vi "Main Page.vi"(8 "error in (no error)":errorcluster, 11 "Node Ptr":T1 format="%.0x") -> (0 "error out":errorcluster)   [LabVIEW 2020, in "Protection and Counter Addon System Explorer.lvlib"]
uses:
  Protection and Counter Addon System Explorer.lvlib
  <vilib>/NI VeriStand/Custom Device API/Custom Device Item Ref.ctl
  <vilib>/NI/NI VeriStand Hardware Resource Discovery/_Types/Filter Type.ctl
  Addon Shared/Types/986x.ctl
  Addon Shared/SubVIs/GUID Lookup.vi
  <vilib>/NI VeriStand/Custom Device API/NI VeriStand - Get Item Property.vi
  <vilib>/NI VeriStand/Custom Device API/Get Item Property (Boolean).vi
  <vilib>/NI VeriStand/Custom Device API/Get Item Property (String).vi
  <vilib>/NI VeriStand/Custom Device API/Get Item Property (Dependent File).vi
  <vilib>/NI VeriStand/Custom Device API/Get Item Property (U32).vi
  <vilib>/NI VeriStand/Custom Device API/Get Item Property (String Array).vi
  <vilib>/NI VeriStand/Custom Device API/Custom Device API.lvlib
  <vilib>/NI/NI VeriStand Hardware Resource Discovery/NIVS Hardware Discovery.lvlib
  Addon Shared/Protection and Counter Addon Shared.lvlib
  SubModules/985x-Support/Source/System Explorer/985x Support System Explorer.lvlib
panel:
  in  "Header":cluster{"Section Name":string}={"Section Name"="Addon Settings"}
  in  "Tab Control":enum32{"Main Setting", "FPGA Settings"}(tab)
  in  "FD ISO Mode":u32(ring) items=["ISO", "Non ISO", "ISO Legacy"]
  in  "Description":string
  in  "Name":string
  out "Version":string
  in  "Port":string
  in  "CAN Browse":bool
  out "XNET Database":refnum<k21>
  out "XNET Cluster":refnum<k21>
  out "I/O Mode":u32(ring) items=["CAN 2.0", "CAN FD", "CAN FD+BRS"]
  in  "Baud Rate":u64
  in  "Termination":enum16{"Off", "On"}(ring)
  in  "FD Baud Rate":u64
  in  "Use Legacy":bool
  in  "Loop Priority":i32=100 format="%.0p"
  in  "985x Chn":u16(ring) caption="Channel Number"
  in  "Use 985x":bool
  in  "Enable Bitfile":bool
  in  "Bitfile Path":path caption="Bitfile Path (Browse the bitfile to check if it supports 985x.)"
  in  "RIO Device":string
  in  "RIO Browse":bool
  in  "SHDocVw.IWebBrowser2":refnum<k7>(container)
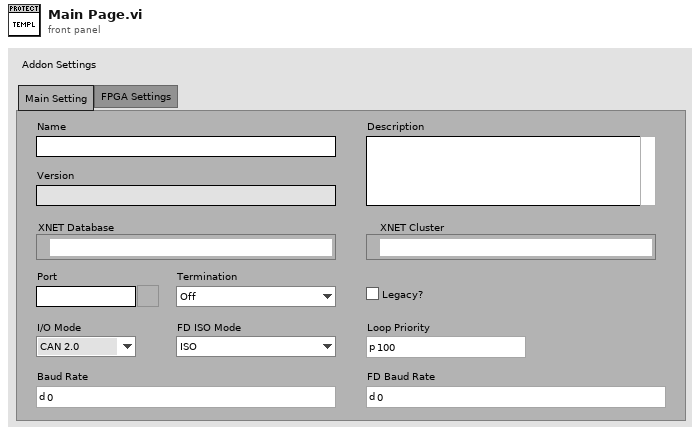
[diagram p1: front panel]
types:
  T1 = typedef "Custom Device API.lvlib/Custom Device Item Ref.ctl" = u64
  T2 = typedef "Protection and Counter Addon Shared.lvlib/986x.ctl" = cluster{"Enable":bool, "RIO Device":string, "Bitfile":path, "985x Valid":bool, "Use 985x":bool, "Channel Number":u32, "Valid Channels":string[]}
  T3 = typedef "Protection and Counter Addon Shared.lvlib/XNET Settings.ctl" = cluster{"Database":refnum<k21>, "Cluster":refnum<k21>, "Port":string, "Baud rate [Bd]":u64, "Termination":u32, "CAN I/O Mode":u32, "FD Baud rate [Bd]":u64, "Priority":i32, "Use Legacy":bool, "FD ISO Mode":u32}
  T4 = typedef "Custom Device API.lvlib/Custom Device Item Info.ctl" = cluster{"Name":string, "Is Channel":bool, "GUID":string, "Is Waveform":bool}
  T5 = typedef "NIVS Hardware Discovery.lvlib/Filter Type.ctl" = enum16{"Device Category", "Product Name", "Ethernet", "XNET", "VISA", "FPGA", "EtherCAT Master", "DAQmx", "GPIB", "Serial"}
  T6 = typedef "Custom Device API.lvlib/Custom Device Commands.ctl" = enum16{"Default", "Item renamed", "Shutdown", "Dynamic button pressed"}
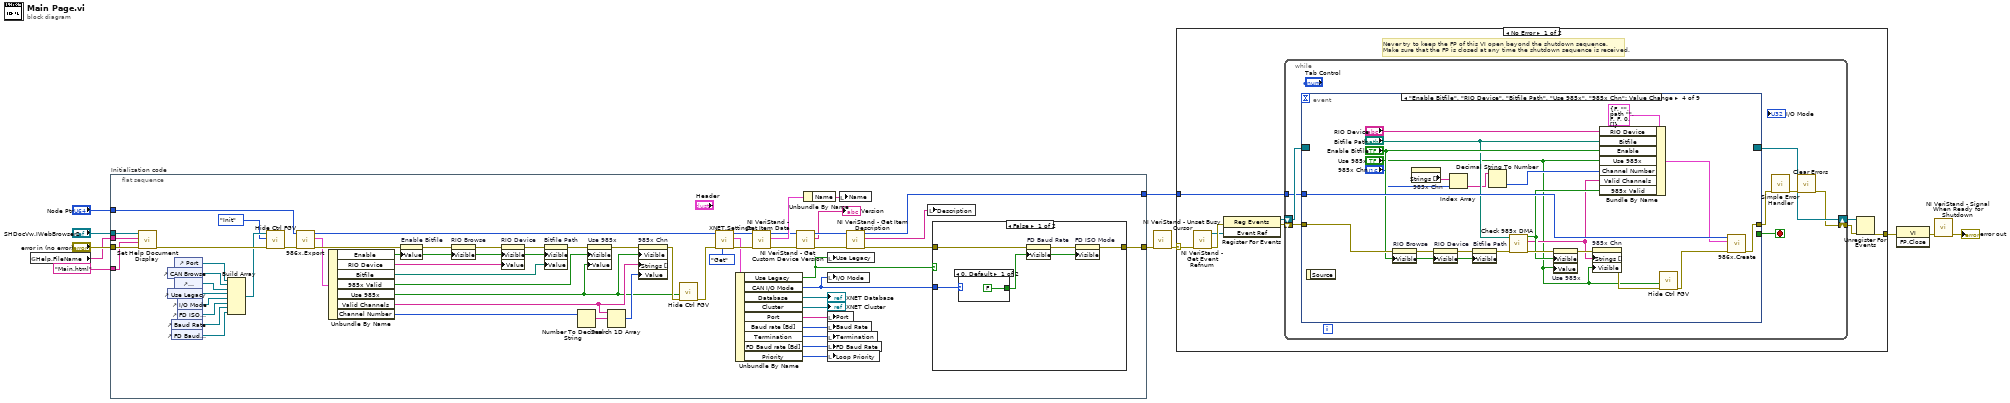
[diagram p0: block diagram]
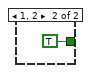
[diagram p2: hidden frame]
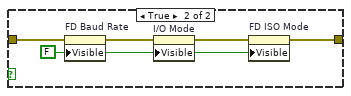
[diagram p3: hidden frame]
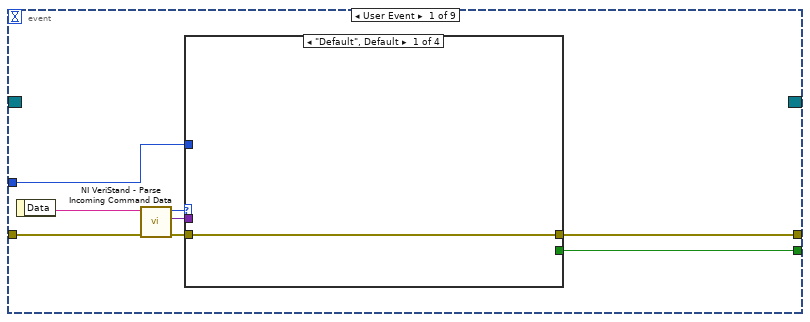
[diagram p4: hidden frame]
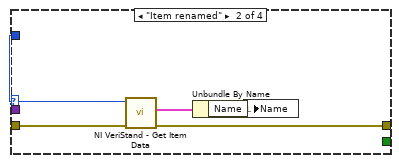
[diagram p5: hidden frame]
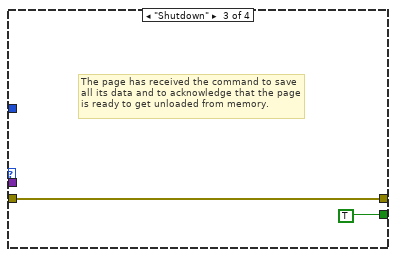
[diagram p6: hidden frame]
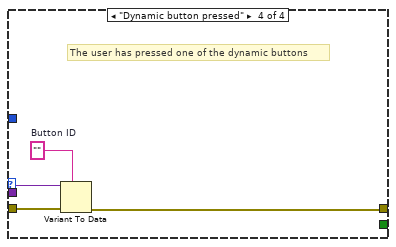
[diagram p7: hidden frame]
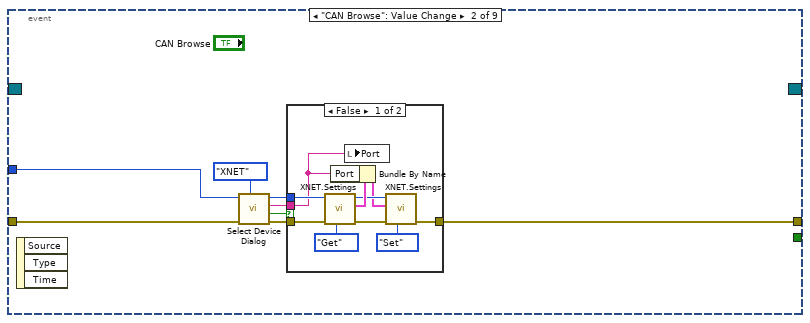
[diagram p8: hidden frame]
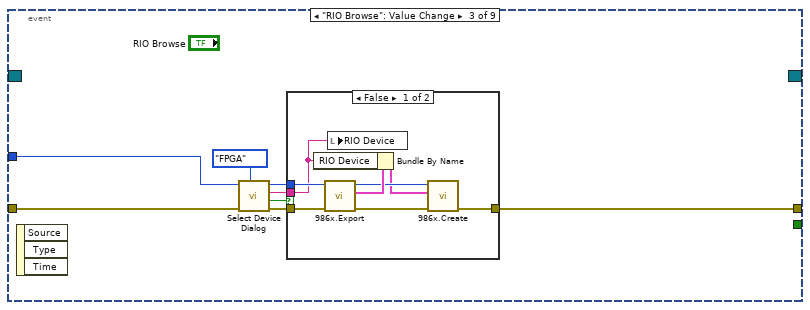
[diagram p10: hidden frame]
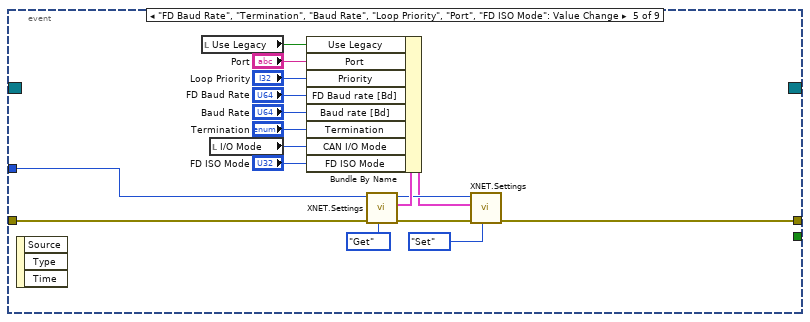
[diagram p12: hidden frame]
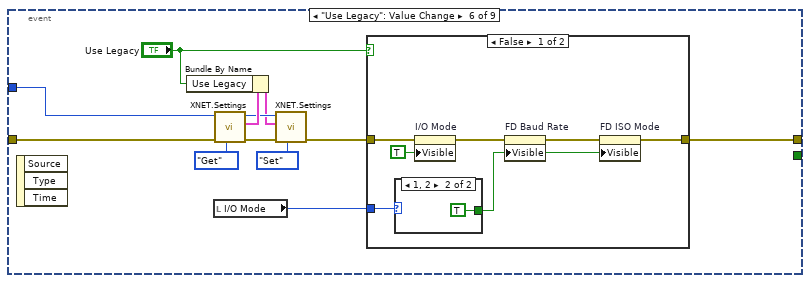
[diagram p13: hidden frame]
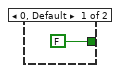
[diagram p14: hidden frame]
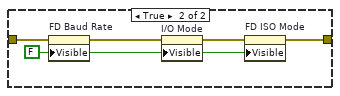
[diagram p15: hidden frame]
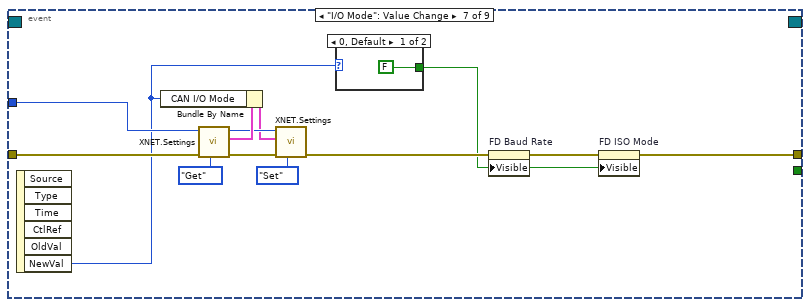
[diagram p16: hidden frame]
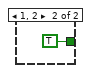
[diagram p17: hidden frame]
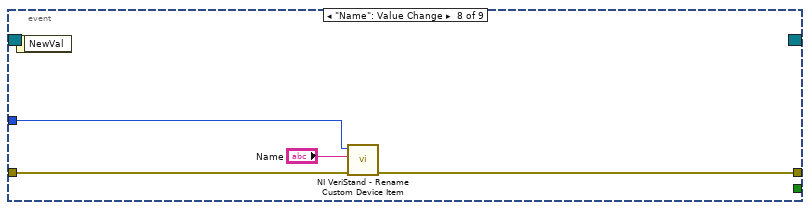
[diagram p18: hidden frame]
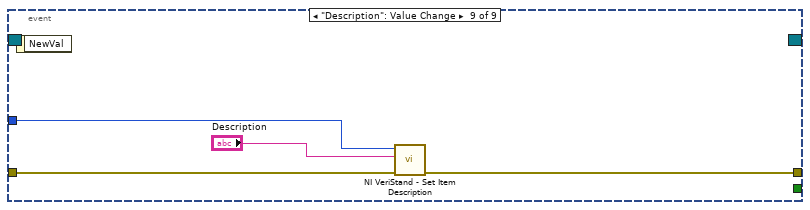
[diagram p19: hidden frame]
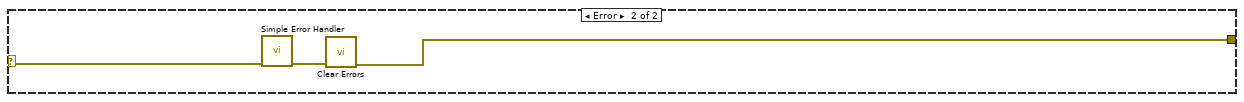
[diagram p20: hidden frame]
diagram:
  n1 = global read "GUID Lookup.vi" "Help.FileName"() -> (w1:string)
  n2 = flat-sequence "Initialization code" {
    tunnel: "error in (no error)" -> [w69]
    tunnel: "Node Ptr" -> [w51]
    tunnel: [w53] -> w7
    tunnel: [w37] -> w4
    tunnel: "SHDocVw.IWebBrowser2" -> [w68]
    tunnel: w1 -> [w67]
    tunnel: "Main.html" ("HTML File") -> [w66]
    frame #0 {
      n3 = call "Set Help Document Display.vi"("error in (no error)"=w69, "HTML File"=w66, "Main CHM File"=w67, "SHDocVw.IWebBrowser2"=w68) -> ("error out"=w20:errorcluster)  [unwired: 7 in]
      n4 = control-ref of="CAN Browse"() -> (w12:refnum<vi>)
      n5 = control-ref of="Use Legacy"() -> (w22:refnum<vi>)
      n6 = control-ref of="Baud Rate"() -> (w25:refnum<vi>)
      n7 = control-ref of="FD Baud Rate"() -> (w26:refnum<vi>)
      n8 = control-ref of="Port"() -> (w13:refnum<vi>)
      n9 = control-ref of="Termination"() -> (w21:refnum<vi>)
      n10 = control-ref of="I/O Mode"() -> (w23:refnum<vi>)
      n11 = control-ref of="FD ISO Mode"() -> (w24:refnum<vi>)
      n12 = Build Array(w13, w12, w21, w22, w23, w24, w25, w26) -> (w18:refnum<vi>[])
      n13 = call "Hide Ctrl FGV.vi"("error in (no error)"=w20, "Action"=enum16{"Init", "Set Visibility"}."Init", "Controls Ref"=w18) -> ("error out"=w19:errorcluster)  [unwired: 8 in]
      n14 = call "986x.Export.vi"("error in (no error)"=w19, "Device Item Ref in"=w51) -> ("error out"=w46:errorcluster, "986x Support"=w45:T2, "Item Ref out"=w50:T1)  [unwired: 7 in]
      n15 = Unbundle By Name(w45) -> ("Enable"=w44:bool, "RIO Device"=w43:string, "Bitfile"=w42:path, "985x Valid"=w32:bool, "Use 985x"=w15:bool, "Valid Channels"=w30:string[], "Channel Number"=w28:u32)
      n16 = property on="Enable Bitfile" class="Bool (strict)"(error in=w46, "Value"=w44) -> (error out=w49:errorcluster)  [unwired: 1 in, 1 out]
      n17 = property on="RIO Browse" class="Bool"(error in=w49, "Visible"=w44) -> (error out=w48:errorcluster)  [unwired: 1 in, 1 out]
      n18 = property on="RIO Device" class="Str"(error in=w48, "Visible"=w44, "Value"=w43) -> (error out=w47:errorcluster)  [unwired: 1 in, 1 out]
      n19 = property on="Bitfile Path" class="Path"(error in=w47, "Visible"=w44, "Value"=w42) -> (error out=w33:errorcluster)  [unwired: 1 in, 1 out]
      n20 = Number To Decimal String(number=w28) -> (decimal integer string=w27:string)  [unwired: 1 in]
      n21 = property on="Use 985x" class="Bool (strict)"(error in=w33, "Visible"=w32, "Value"=w15) -> (error out=w31:errorcluster)  [unwired: 1 in, 1 out]
      n22 = Search 1D Array(1D array=w30, element=w27) -> (index of element=w29:i32)  [unwired: 1 in]
      n23 = property on="985x Chn" class="Ring (strict)"(error in=w31, "Visible"=w15, "Strings []"=w30, "Value"=w29) -> (error out=w16:errorcluster)  [unwired: 1 in, 1 out]
      n24 = call "Hide Ctrl FGV.vi"("error in (no error)"=w16, "Hide"=w15) -> ("error out"=w14:errorcluster)  [unwired: 9 in]
      n25 = call "XNET.Settings.vi"("Action"=enum8{"Get", "Set"}."Get", "error in (no error)"=w14, "Parent Ref in"=w50) -> ("error out"=w65:errorcluster, "XNET Settings"=w62:T3, "Item Ref out"=w64:T1)  [unwired: 6 in]
      n26 = Unbundle By Name(w62) -> ("Use Legacy"=w54:bool, "CAN I/O Mode"=w52:u32, "Database"=→"XNET Database":refnum<k21>, "Cluster"=→"XNET Cluster":refnum<k21>, "Port"=w59:string, "Baud rate [Bd]"=w58:u64, "Termination"=w57:u32, "FD Baud rate [Bd]"=w56:u64, "Priority"=w55:i32)
      n27 = call <vilib>:"NI VeriStand - Get Item Data.vi"("error in (no error)"=w65, "Item Ref in"=w64) -> ("error out"=w41:errorcluster, "Item Info"=w71:T4, "Item Ref out"=w40:T1)  [unwired: 7 out]
      n28 = call <vilib>:"NI VeriStand - Get Custom Device Version.vi"("error in (no error)"=w41, "Device Ref in"=w40) -> ("error out"=w36:errorcluster, "Value"=→"Version":string, "Device Ref out"=w39:T1)  [unwired: 7 in]
      n29 = Unbundle By Name(w71) -> ("Name"=w70:string)
      n30 = local write "Use Legacy"(w54) -> ()
      n31 = local write "I/O Mode"(w52) -> ()
      n32 = local write "Port"(w59) -> ()
      n33 = local write "Baud Rate"(w58) -> ()
      n34 = local write "Termination"(w57) -> ()
      n35 = local write "FD Baud Rate"(w56) -> ()
      n36 = local write "Loop Priority"(w55) -> ()
      n37 = local write "Name"(w70) -> ()
      n38 = call <vilib>:"NI VeriStand - Get Item Description.vi"("error in (no error)"=w36, "Item Ref in"=w39) -> ("error out"=w35:errorcluster, "Description"=w34:string, "Item Ref out"=w37:T1)  [unwired: 6 in, 1 out]
      n39 = local write "Description"(w34) -> ()
      n40 = case shown="False" w54 {
        tunnel: w35 -> [w75 w82]
        tunnel: [w73 w80] -> w53
        tunnel: w52 -> [w76 _]
        frame False {
          n41 = case shown="0, Default" w76 {
            tunnel: [FALSE TRUE] -> w72
            frame 0, Default {
            }
            frame 1, 2 {
            }
          }
          n42 = property on="FD Baud Rate" class="DigNum (strict)"(error in=w75, "Visible"=w72) -> (error out=w74:errorcluster)  [unwired: 1 in, 1 out]
          n43 = property on="FD ISO Mode" class="Ring (strict)"(error in=w74, "Visible"=w72) -> (error out=w73:errorcluster)  [unwired: 1 in, 1 out]
        }
        frame True {
          w79 = FALSE ("Visible")
          n44 = property on="FD Baud Rate" class="DigNum (strict)"(error in=w82, "Visible"=w79) -> (error out=w83:errorcluster)  [unwired: 1 in, 1 out]
          n45 = property on="I/O Mode" class="Ring (strict)"(error in=w83, "Visible"=w79) -> (error out=w81:errorcluster)  [unwired: 1 in, 1 out]
          n46 = property on="FD ISO Mode" class="Ring (strict)"(error in=w81, "Visible"=w79) -> (error out=w80:errorcluster)  [unwired: 1 in, 1 out]
        }
      }
    }
  }
  n47 = call <vilib>:"NI VeriStand - Unset Busy Cursor.vi"("error in (no error)"=w7) -> ("error out"=w6:errorcluster)  [unwired: 10 out]
  n48 = case shown="No Error" w6 {
    selector: w6 -> [w84 w247]
    tunnel: [w89 w245] -> w11
    tunnel: w4 -> [w85 _]
    frame No Error {
      # "Never try to keep the FP of this VI open beyond the shutdown sequence.\nMake sure that the FP is closed at any time the shutdown sequence is received."
      n49 = call <vilib>:"NI VeriStand - Get Event Refnum.vi"("error in (no error)"=w84) -> ("error out"=w92:errorcluster, "Event Ref"=w88:refnum<user-event>)  [unwired: 9 out]
      n50 = register-events(error in=w92, w88) -> (reference out=w86:refnum<event-registration>, error out=w87:errorcluster)  [unwired: 1 in]
      n51 = while {
        tunnel: w85 -> [w96]
        shift-right: [w93] -> w90
        shift-left: w87 -> [w99]
        shift-right: [w100] -> w91
        shift-left: w86 -> [w98]
        stop <- w97 stop-if-true
        n52 = event shown="[3] \"Enable Bitfile\", \"RIO Device\", \"Bitfile Path\", \"Use 985x\", \"985x Chn\": Value Change" {
          selector: w98 -> [_ _ _ _ _ _ _ _ _]
          dyn-events: [_ _ _ _ _ _ _ _ _] -> w100
          timeout: _ -> [_ _ _ _ _ _ _ _ _]
          tunnel: w99 -> [w108 w123 w142 w175 w189 w201 w228 w240 w244]
          tunnel: [w104 _ _ _ _ _ _ _ _] -> w97
          tunnel: [w103 w121 w140 w178 w188 w197 w223 w239 w243] -> w95
          tunnel: w96 -> [w102 w122 w141 w174 w187 w200 w227 w238 w242]
          event User Event {
            n53 = event-data() -> ("Data"=w107:string)  [unwired: 1 out]
            n54 = call <vilib>:"NI VeriStand - Parse Incoming Command Data.vi"("error in (no error)"=w108, "Incoming data"=w107) -> ("error out"=w106:errorcluster, "Outgoing data"=w101:variant, "Action"=w105:T6)  [unwired: 7 out]
            n55 = case shown="\"Default\", Default" w105 {
              tunnel: w106 -> [w109 w114 w115 w120]
              tunnel: [_ _ TRUE _] -> w104
              tunnel: [w109 w111 w115 w117] -> w103
              tunnel: w102 -> [_ w113 _ _]
              tunnel: w101 -> [_ _ _ w119]
              frame "Default", Default {
              }
              frame "Item renamed" {
                n56 = call <vilib>:"NI VeriStand - Get Item Data.vi"("error in (no error)"=w114, "Item Ref in"=w113) -> ("error out"=w111:errorcluster, "Item Info"=w112:T4)  [unwired: 8 out]
                n57 = Unbundle By Name(w112) -> ("Name"=w110:string)
                n58 = local write "Name"(w110) -> ()
              }
              frame "Shutdown" {
                # "The page has received the command to save all its data and to acknowledge that the page is ready to get unloaded from memory."
              }
              frame "Dynamic button pressed" {
                w118 = ""  # Button ID
                # "The user has pressed one of the dynamic buttons"
                n59 = Variant To Data(error in=w120, type=w118, Variant=w119) -> (error out=w117:errorcluster)  [unwired: 1 out]
              }
            }
          }
          event "CAN Browse": Value Change {
            n60 = event-data() -> ()  [unwired: 4 out]
            n61 = call <vilib>:"Select Device Dialog.vi"("Filter Type"=Filter_Type."XNET", "error in (no error)"=w123, "Item Ref in"=w122) -> ("error out"=w127:errorcluster, "Cancelled?"=w126:bool, "Selected Alias"=w125:string, "Item Ref out"=w128:T1)  [unwired: 5 in]
            n62 = case shown="False" w126 {
              tunnel: w128 -> [w136 _]
              tunnel: [w133 w139] -> w121
              tunnel: w127 -> [w130 w139]
              tunnel: w125 -> [w129 _]
              frame False {
                n63 = call "XNET.Settings.vi"("Action"=enum8{"Get", "Set"}."Get", "error in (no error)"=w130, "Parent Ref in"=w136) -> ("error out"=w131:errorcluster, "XNET Settings"=w137:T3, "Item Ref out"=w134:T1)  [unwired: 6 in]
                n64 = Bundle By Name(cluster=w137, "Port"=w129) -> (w132:T3)
                n65 = local write "Port"(w129) -> ()
                n66 = call "XNET.Settings.vi"("Action"=enum8{"Get", "Set"}."Set", "error in (no error)"=w131, "XNET Settings"=w132, "Parent Ref in"=w134) -> ("error out"=w133:errorcluster)  [unwired: 5 in, 2 out]
              }
              frame True {
              }
            }
          }
          event "RIO Browse": Value Change {
            n67 = event-data() -> ()  [unwired: 4 out]
            n68 = call <vilib>:"Select Device Dialog.vi"("Filter Type"=Filter_Type."FPGA", "error in (no error)"=w142, "Item Ref in"=w141) -> ("error out"=w146:errorcluster, "Cancelled?"=w145:bool, "Selected Alias"=w144:string, "Item Ref out"=w147:T1)  [unwired: 5 in]
            n69 = case shown="False" w145 {
              tunnel: w147 -> [w154 _]
              tunnel: [w149 w156] -> w140
              tunnel: w146 -> [w153 w156]
              tunnel: w144 -> [w152 _]
              frame False {
                n70 = call "986x.Export.vi"("error in (no error)"=w153, "Device Item Ref in"=w154) -> ("error out"=w151:errorcluster, "986x Support"=w155:T2, "Item Ref out"=w150:T1)  [unwired: 7 in]
                n71 = Bundle By Name(cluster=w155, "RIO Device"=w152) -> (w148:T2)
                n72 = local write "RIO Device"(w152) -> ()
                n73 = call "986x.Create.vi"("error in (no error)"=w151, "986x Support"=w148, "Device Item Ref in"=w150) -> ("error out"=w149:errorcluster)  [unwired: 7 in, 1 out]
              }
              frame True {
              }
            }
          }
          event "Enable Bitfile", "RIO Device", "Bitfile Path", "Use 985x", "985x Chn": Value Change {
            n74 = event-data() -> ()  [unwired: 2 out]
            n75 = property on="RIO Browse" class="Bool"(error in=w175, "Visible"="Enable Bitfile") -> (error out=w176:errorcluster)  [unwired: 1 in, 1 out]
            n76 = property on="985x Chn" class="Ring (strict)"() -> ("Strings []"=w164:string[])  [unwired: 2 in, 2 out]
            n77 = property on="RIO Device" class="Str"(error in=w176, "Visible"="Enable Bitfile") -> (error out=w177:errorcluster)  [unwired: 1 in, 1 out]
            n78 = Index Array(array=w164, index="985x Chn") -> (element=w161:string)
            n79 = property on="Bitfile Path" class="Path"(error in=w177, "Visible"="Enable Bitfile") -> (error out=w168:errorcluster)  [unwired: 1 in, 1 out]
            n80 = Decimal String To Number(string=w161) -> (number=w160:i32)  [unwired: 2 in, 1 out]
            n81 = call "Check 985x DMA.vi"("error in (no error)"=w168, "Bitfile path"="Bitfile Path") -> ("error out"=w167:errorcluster, "Available Channels"=w162:string[], "Found"=w166:bool)  [unwired: 7 in]
            n82 = property on="Use 985x" class="Bool (strict)"(error in=w167, "Visible"=w166, "Value"="Use 985x") -> (error out=w165:errorcluster)  [unwired: 1 in, 1 out]
            n83 = property on="985x Chn" class="Ring (strict)"(error in=w165, "Strings []"=w162, "Visible"="Use 985x") -> (error out=w159:errorcluster)  [unwired: 1 in, 1 out]
            n84 = Bundle By Name(cluster=T2 {"Enable"=FALSE, "RIO Device"="", "Bitfile"=path "", "985x Valid"=FALSE, "Use 985x"=FALSE, "Channel Number"=0, "Valid Channels"=[]} ("986x Support"), "RIO Device"="RIO Device", "Bitfile"="Bitfile Path", "Enable"="Enable Bitfile", "Use 985x"="Use 985x", "Channel Number"=w160, "Valid Channels"=w162, "985x Valid"=w166) -> (w172:T2)
            n85 = call "Hide Ctrl FGV.vi"("error in (no error)"=w159, "Hide"="Use 985x") -> ("error out"=w158:errorcluster)  [unwired: 9 in]
            n86 = call "986x.Create.vi"("error in (no error)"=w158, "986x Support"=w172, "Device Item Ref in"=w174) -> ("error out"=w178:errorcluster)  [unwired: 7 in, 1 out]
          }
          event "FD Baud Rate", "Termination", "Baud Rate", "Loop Priority", "Port", "FD ISO Mode": Value Change {
            n87 = event-data() -> ()  [unwired: 4 out]
            n88 = local read "Use Legacy"() -> (w181:bool)
            n89 = local read "I/O Mode"() -> (w180:u32)
            n90 = call "XNET.Settings.vi"("Action"=enum8{"Get", "Set"}."Get", "error in (no error)"=w189, "Parent Ref in"=w187) -> ("error out"=w190:errorcluster, "XNET Settings"=w194:T3, "Item Ref out"=w192:T1)  [unwired: 6 in]
            n91 = Bundle By Name(cluster=w194, "Use Legacy"=w181, "Port"="Port", "Priority"="Loop Priority", "FD Baud rate [Bd]"="FD Baud Rate", "Baud rate [Bd]"="Baud Rate", "Termination"="Termination", "CAN I/O Mode"=w180, "FD ISO Mode"="FD ISO Mode") -> (w191:T3)
            n92 = call "XNET.Settings.vi"("Action"=enum8{"Get", "Set"}."Set", "error in (no error)"=w190, "XNET Settings"=w191, "Parent Ref in"=w192) -> ("error out"=w188:errorcluster)  [unwired: 5 in, 2 out]
          }
          event "Use Legacy": Value Change {
            n93 = event-data() -> ()  [unwired: 4 out]
            n94 = local read "I/O Mode"() -> (w196:u32)
            n95 = call "XNET.Settings.vi"("Action"=enum8{"Get", "Set"}."Get", "error in (no error)"=w201, "Parent Ref in"=w200) -> ("error out"=w202:errorcluster, "XNET Settings"=w206:T3, "Item Ref out"=w204:T1)  [unwired: 6 in]
            n96 = Bundle By Name(cluster=w206, "Use Legacy"="Use Legacy") -> (w203:T3)
            n97 = call "XNET.Settings.vi"("Action"=enum8{"Get", "Set"}."Set", "error in (no error)"=w202, "XNET Settings"=w203, "Parent Ref in"=w204) -> ("error out"=w198:errorcluster)  [unwired: 5 in, 2 out]
            n98 = case shown="False" "Use Legacy" {
              tunnel: w198 -> [w213 w220]
              tunnel: [w209 w218] -> w197
              tunnel: w196 -> [w214 _]
              frame False {
                n99 = case shown="1, 2" w214 {
                  tunnel: [FALSE TRUE] -> w208
                  frame 0, Default {
                  }
                  frame 1, 2 {
                  }
                }
                n100 = property on="I/O Mode" class="Ring (strict)"(error in=w213, "Visible"=TRUE) -> (error out=w212:errorcluster)  [unwired: 1 in, 1 out]
                n101 = property on="FD Baud Rate" class="DigNum (strict)"(error in=w212, "Visible"=w208) -> (error out=w210:errorcluster)  [unwired: 1 in, 1 out]
                n102 = property on="FD ISO Mode" class="Ring (strict)"(error in=w210, "Visible"=w208) -> (error out=w209:errorcluster)  [unwired: 1 in, 1 out]
              }
              frame True {
                w217 = FALSE ("Visible")
                n103 = property on="FD Baud Rate" class="DigNum (strict)"(error in=w220, "Visible"=w217) -> (error out=w221:errorcluster)  [unwired: 1 in, 1 out]
                n104 = property on="I/O Mode" class="Ring (strict)"(error in=w221, "Visible"=w217) -> (error out=w219:errorcluster)  [unwired: 1 in, 1 out]
                n105 = property on="FD ISO Mode" class="Ring (strict)"(error in=w219, "Visible"=w217) -> (error out=w218:errorcluster)  [unwired: 1 in, 1 out]
              }
            }
          }
          event "I/O Mode": Value Change {
            n106 = event-data() -> ("NewVal"=w225:u32)  [unwired: 6 out]
            n107 = call "XNET.Settings.vi"("Action"=enum8{"Get", "Set"}."Get", "error in (no error)"=w228, "Parent Ref in"=w227) -> ("error out"=w229:errorcluster, "XNET Settings"=w233:T3, "Item Ref out"=w231:T1)  [unwired: 6 in]
            n108 = Bundle By Name(cluster=w233, "CAN I/O Mode"=w225) -> (w230:T3)
            n109 = call "XNET.Settings.vi"("Action"=enum8{"Get", "Set"}."Set", "error in (no error)"=w229, "XNET Settings"=w230, "Parent Ref in"=w231) -> ("error out"=w226:errorcluster)  [unwired: 5 in, 2 out]
            n110 = case shown="0, Default" w225 {
              tunnel: [FALSE TRUE] -> w222
              frame 0, Default {
              }
              frame 1, 2 {
              }
            }
            n111 = property on="FD Baud Rate" class="DigNum (strict)"(error in=w226, "Visible"=w222) -> (error out=w224:errorcluster)  [unwired: 1 in, 1 out]
            n112 = property on="FD ISO Mode" class="Ring (strict)"(error in=w224, "Visible"=w222) -> (error out=w223:errorcluster)  [unwired: 1 in, 1 out]
          }
          event "Name": Value Change {
            n113 = event-data() -> ()  [unwired: 2 out]
            n114 = call <vilib>:"NI VeriStand - Rename Custom Device Item.vi"("error in (no error)"=w240, "New Name"="Name", "Item Ref in"=w238) -> ("error out"=w239:errorcluster)  [unwired: 1 in, 7 out]
          }
          event "Description": Value Change {
            n115 = event-data() -> ()  [unwired: 2 out]
            n116 = call <vilib>:"NI VeriStand - Set Item Description.vi"("error in (no error)"=w244, "Description"="Description", "Item Ref in"=w242) -> ("error out"=w243:errorcluster)  [unwired: 6 in, 2 out]
          }
        }
        n117 = call <vilib>:"Simple Error Handler.vi"("error in (no error)"=w95) -> ("error out"=w94:errorcluster)  [unwired: 1 in, 7 out]
        n118 = call <vilib>:"Clear Errors.vi"("error in (no error)"=w94) -> ("error out"=w93:errorcluster)  [unwired: 1 in, 5 out]
      }
      n119 = Unregister For Events(event registration refnum=w91, error in=w90) -> (error out=w89:errorcluster)
    }
    frame Error {
      n120 = call <vilib>:"Simple Error Handler.vi"("error in (no error)"=w247) -> ("error out"=w246:errorcluster)  [unwired: 1 in, 7 out]
      n121 = call <vilib>:"Clear Errors.vi"("error in (no error)"=w246) -> ("error out"=w245:errorcluster)  [unwired: 1 in, 5 out]
    }
  }
  n122 = invoke class="VI" method="FP.Close"(error in=w11) -> (error out=w10:errorcluster)  [unwired: 2 in, 2 out]
  n123 = call <vilib>:"NI VeriStand - Signal When Ready for Shutdown.vi"("error in (no error)"=w10) -> ("error out"=→"error out":errorcluster)  [unwired: 10 out]
